vi "质控数据存储(子VI).vi"(4 "CODMn":refnum<vi>, 6 "总磷":refnum<vi>, 7 "CODCr":refnum<vi>, 10 "氨氮":refnum<vi>, 11 "总氮":refnum<vi>) -> ()   [LabVIEW 2016, in "质控单元.lvlib"]
uses:
  <vilib>/ptbypt/NI_PtbyPt.lvlib
panel:
  out "columns":string[](array[string])
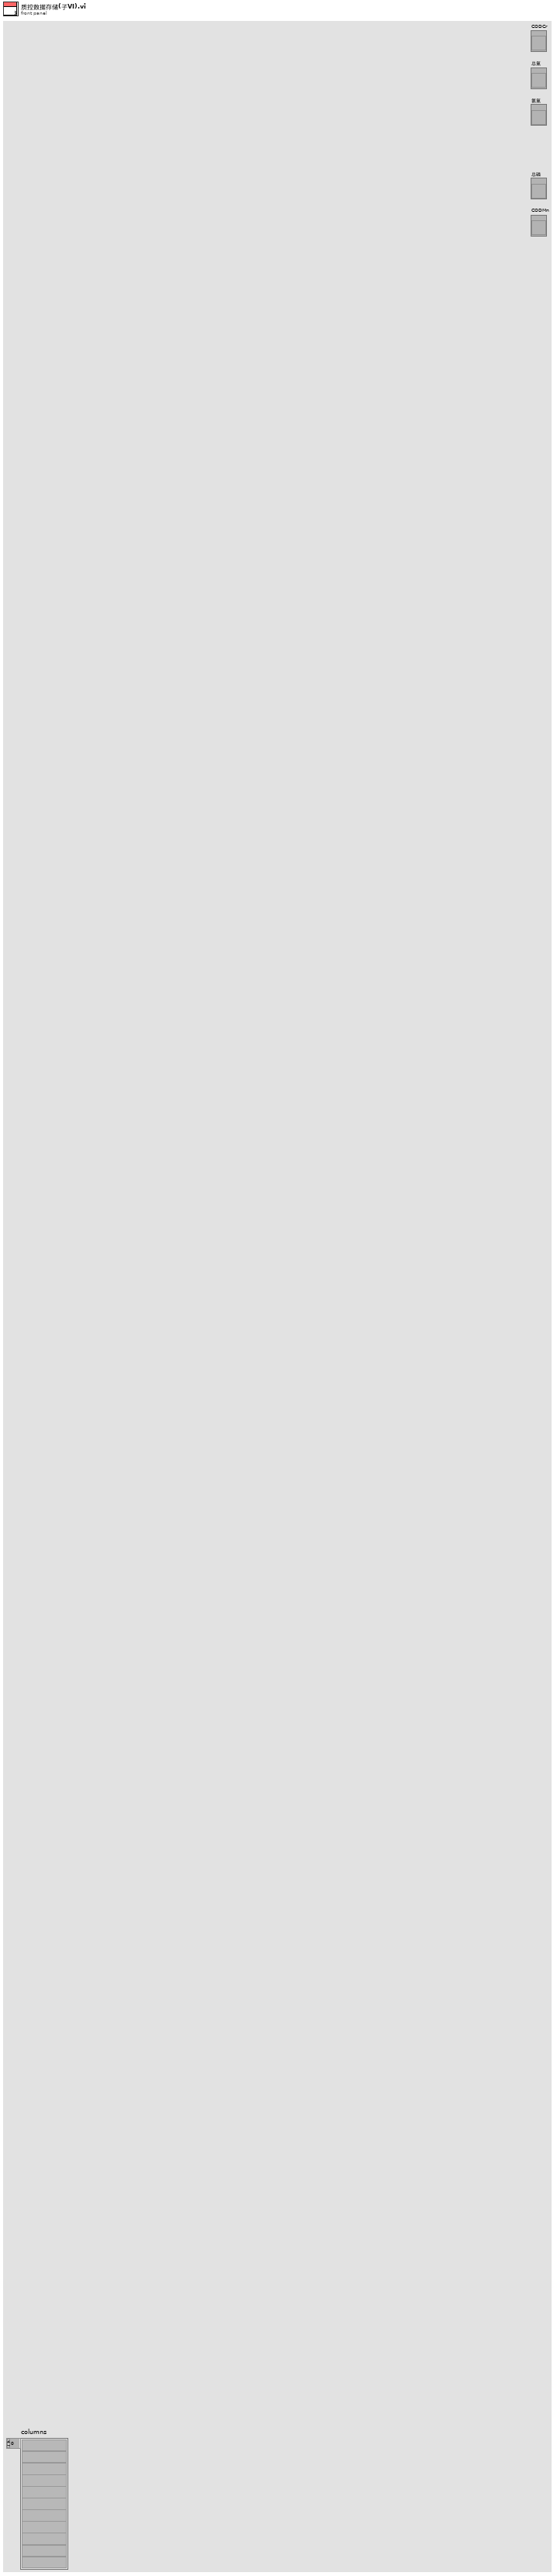
[diagram p1: front panel]
types:
  T1 = cluster{"时间":timestamp, "参数":string, "加标前水样测试时间":timestamp, "加标前水样浓度值（mg/L)":sgl, "加标后水样浓度值（mg/L)":sgl, "加标母液浓度值（mg/L)":sgl, "加标体积":dbl, "加标水杯定容体积":dbl, "加标回收率":dbl}
  T2 = cluster{"因子编码":u32, "单位":u16, "标样参考值":sgl, "水样数据时间":timestamp, "水样实测值":sgl, "水样数据标识":string, "标样数据时间":timestamp, "标样实测值":sgl, "标样数据标识":string, "空白数据时间":timestamp, "空白实测值":sgl, "空白数据标识":string, "零点核查数据时间":timestamp, "零点核查实测值":sgl, "零点核查数据标识":string, "跨度核查数据时间":timestamp, "跨度核查实测值":sgl, "跨度核查数据标识":string, "加标回收数据时间":timestamp, "加标回收实测值":sgl, "加标回收数据标识":string, "平行样数据时间":timestamp, "平行样实测值":sgl, "平行样数据标识":string}
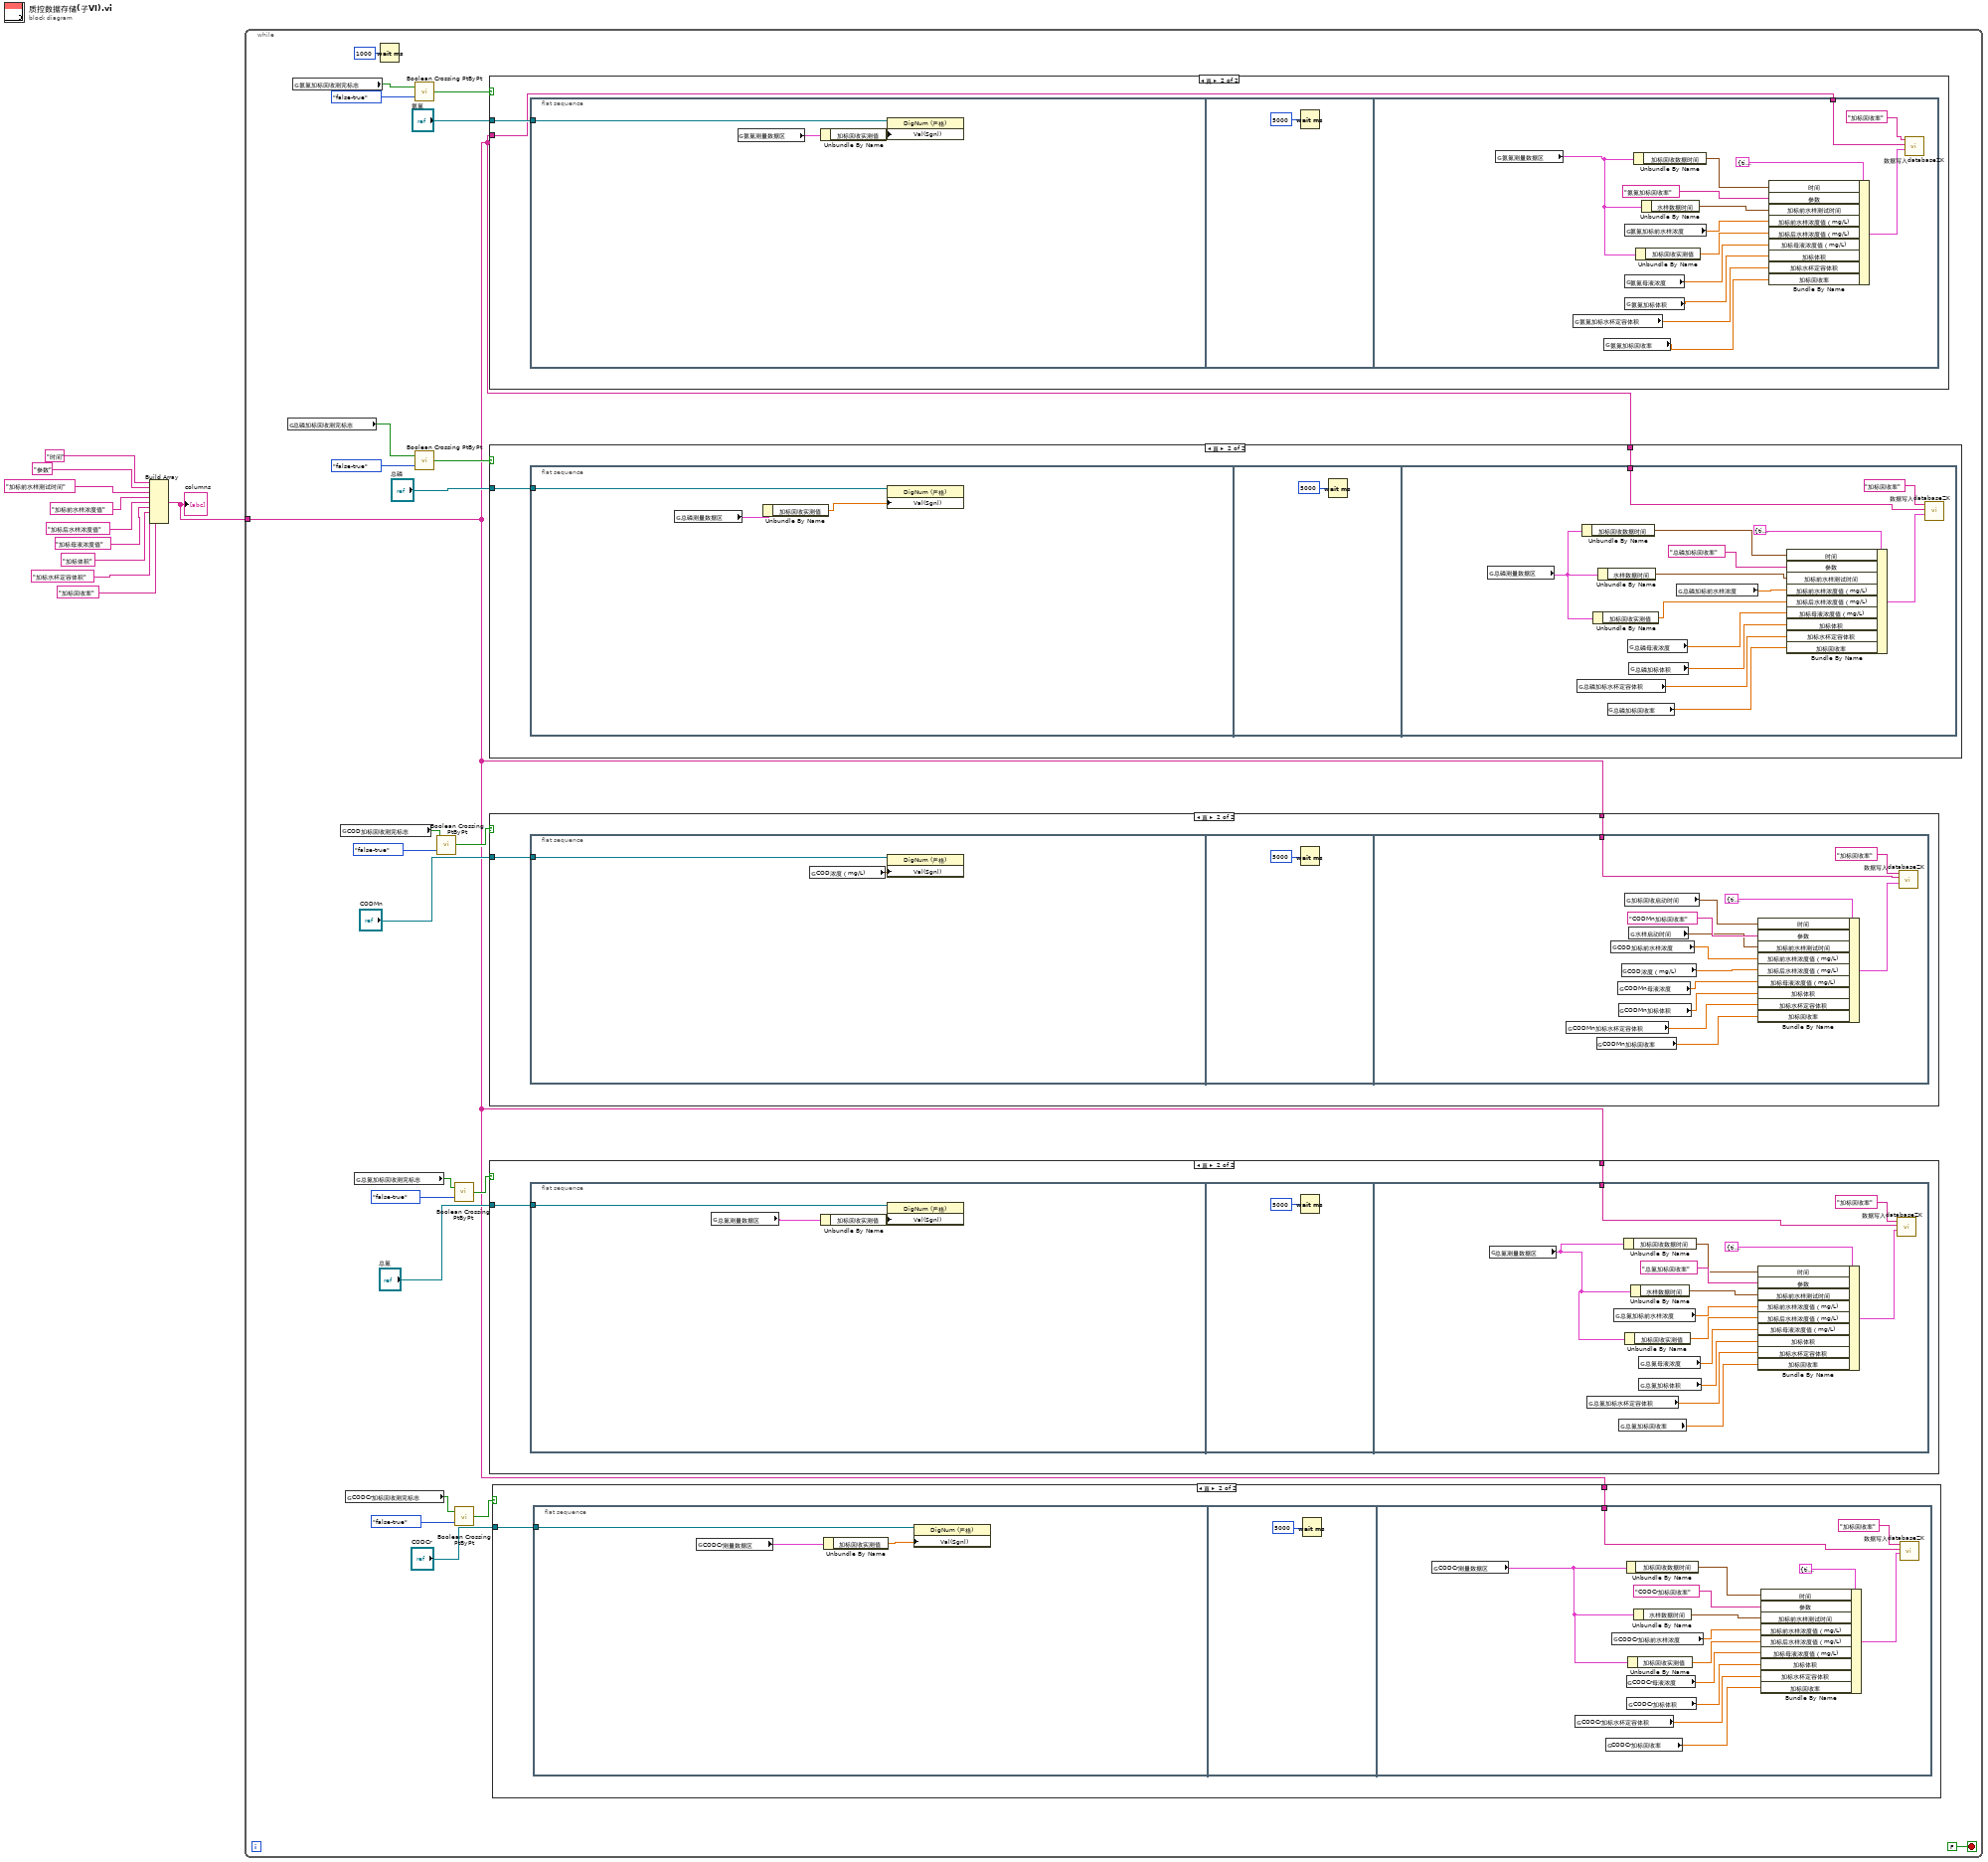
[diagram p0: block diagram]
diagram:
  n1 = Build Array("时间" ("table"), "参数" ("table"), "加标前水样测试时间" ("table"), "加标前水样浓度值" ("元素"), "加标后水样浓度值" ("元素"), "加标母液浓度值" ("元素"), "加标体积" ("元素"), "加标水杯定容体积" ("元素"), "加标回收率" ("元素")) -> (w1:string[])
  "columns" <- w1
  n2 = while {
    tunnel: w1 -> [w11]
    stop <- FALSE stop-if-true
    n3 = global read "质控测完标志全局 1.vi" "总磷加标回收测完标志"() -> (w24:bool)
    n4 = global read "质控测完标志全局 1.vi" "氨氮加标回收测完标志"() -> (w19:bool)
    n5 = global read "质控测完标志全局 1.vi" "COD加标回收测完标志"() -> (w26:bool)
    n6 = global read "质控测完标志全局 1.vi" "CODCr加标回收测完标志"() -> (w32:bool)
    n7 = global read "质控测完标志全局 1.vi" "总氮加标回收测完标志"() -> (w29:bool)
    n8 = Wait (ms)(milliseconds to wait=u32 1000 ("等待时间（毫秒）")) -> ()  [unwired: 1 out]
    n9 = call <vilib>:"Boolean Crossing PtByPt.vi"("direction"=enum16{"either", "false-true", "true-false"}."false-true", "input"=w19) -> ("crossing"=w20:bool)  [unwired: 1 in]
    n10 = call <vilib>:"Boolean Crossing PtByPt.vi"("direction"=enum16{"either", "false-true", "true-false"}."false-true", "input"=w24) -> ("crossing"=w23:bool)  [unwired: 1 in]
    n11 = call <vilib>:"Boolean Crossing PtByPt.vi"("direction"=enum16{"either", "false-true", "true-false"}."false-true", "input"=w26) -> ("crossing"=w27:bool)  [unwired: 1 in]
    n12 = call <vilib>:"Boolean Crossing PtByPt.vi"("direction"=enum16{"either", "false-true", "true-false"}."false-true", "input"=w29) -> ("crossing"=w30:bool)  [unwired: 1 in]
    n13 = call <vilib>:"Boolean Crossing PtByPt.vi"("direction"=enum16{"either", "false-true", "true-false"}."false-true", "input"=w32) -> ("crossing"=w33:bool)  [unwired: 1 in]
    n14 = case shown="真" w20 {
      tunnel: "氨氮" -> [_ w113]
      tunnel: w11 -> [_ w112]
      frame False {
      }
      frame True {
        n15 = flat-sequence {
          tunnel: w113 -> [w114]
          tunnel: w112 -> [w118]
          frame #0 {
            n16 = global read "与氨氮交互全局.vi" "氨氮测量数据区"() -> (w115:T2)
            n17 = Unbundle By Name(w115) -> ("加标回收实测值"=w116:sgl)
            n18 = property on="属性节点" class="DigNum (严格)"(reference=w114, "Val(Sgnl)"=w116) -> ()  [unwired: 1 in, 2 out]
          }
          frame #1 {
            n19 = Wait (ms)(milliseconds to wait=u32 5000 ("等待时间（毫秒）")) -> ()  [unwired: 1 out]
          }
          frame #2 {
            n20 = global read "与氨氮交互全局.vi" "氨氮测量数据区"() -> (w125:T2)
            n21 = global read "加标回收状态全局变量.vi" "氨氮加标水杯定容体积"() -> (w121:dbl)
            n22 = global read "加标回收状态全局变量.vi" "氨氮加标回收率"() -> (w122:dbl)
            n23 = global read "水样浓度全局.vi" "氨氮加标前水样浓度"() -> (w131:dbl)
            n24 = global read "加标回收状态全局变量.vi" "氨氮母液浓度"() -> (w119:dbl)
            n25 = global read "加标回收状态全局变量.vi" "氨氮加标体积"() -> (w120:dbl)
            n26 = Unbundle By Name(w125) -> ("加标回收数据时间"=w128:timestamp)
            n27 = Unbundle By Name(w125) -> ("加标回收实测值"=w130:sgl)
            n28 = Unbundle By Name(w125) -> ("水样数据时间"=w126:timestamp)
            n29 = Bundle By Name(cluster=T1 {"时间"=timestamp(0 s since 1904-01-01), "参数"="", "加标前水样测试时间"=timestamp(0 s since 1904-01-01), "加标前水样浓度值（mg/L)"=0.0, "加标后水样浓度值（mg/L)"=0.0, "加标母液浓度值（mg/L)"=0.0, "加标体积"=0.0, "加标水杯定容体积"=0.0, "加标回收率"=0.0} ("data"), "时间"=w128, "参数"="氨氮加标回收率" ("table"), "加标前水样测试时间"=w126, "加标前水样浓度值（mg/L)"=w131, "加标后水样浓度值（mg/L)"=w130, "加标母液浓度值（mg/L)"=w119, "加标体积"=w120, "加标水杯定容体积"=w121, "加标回收率"=w122) -> (w123:T1)
            n30 = call "数据写入databaseZK.vi"("data"=w123, "columns"=w118, "table"="加标回收率") -> ()  [unwired: 8 in, 1 out]
          }
        }
      }
    }
    n31 = case shown="真" w23 {
      tunnel: "总磷" -> [_ w93]
      tunnel: w11 -> [_ w92]
      frame False {
      }
      frame True {
        n32 = flat-sequence {
          tunnel: w93 -> [w94]
          tunnel: w92 -> [w98]
          frame #0 {
            n33 = global read "与总磷交互全局.vi" "总磷测量数据区"() -> (w95:T2)
            n34 = Unbundle By Name(w95) -> ("加标回收实测值"=w96:sgl)
            n35 = property on="属性节点" class="DigNum (严格)"(reference=w94, "Val(Sgnl)"=w96) -> ()  [unwired: 1 in, 2 out]
          }
          frame #1 {
            n36 = Wait (ms)(milliseconds to wait=u32 5000 ("等待时间（毫秒）")) -> ()  [unwired: 1 out]
          }
          frame #2 {
            n37 = global read "与总磷交互全局.vi" "总磷测量数据区"() -> (w105:T2)
            n38 = global read "加标回收状态全局变量.vi" "总磷加标水杯定容体积"() -> (w100:dbl)
            n39 = Unbundle By Name(w105) -> ("加标回收数据时间"=w108:timestamp)
            n40 = Unbundle By Name(w105) -> ("加标回收实测值"=w106:sgl)
            n41 = Unbundle By Name(w105) -> ("水样数据时间"=w107:timestamp)
            n42 = global read "加标回收状态全局变量.vi" "总磷加标回收率"() -> (w99:dbl)
            n43 = global read "加标回收状态全局变量.vi" "总磷母液浓度"() -> (w102:dbl)
            n44 = global read "加标回收状态全局变量.vi" "总磷加标体积"() -> (w101:dbl)
            n45 = global read "水样浓度全局.vi" "总磷加标前水样浓度"() -> (w111:dbl)
            n46 = Bundle By Name(cluster=T1 {"时间"=timestamp(0 s since 1904-01-01), "参数"="", "加标前水样测试时间"=timestamp(0 s since 1904-01-01), "加标前水样浓度值（mg/L)"=0.0, "加标后水样浓度值（mg/L)"=0.0, "加标母液浓度值（mg/L)"=0.0, "加标体积"=0.0, "加标水杯定容体积"=0.0, "加标回收率"=0.0} ("data"), "时间"=w108, "参数"="总磷加标回收率" ("table"), "加标前水样测试时间"=w107, "加标前水样浓度值（mg/L)"=w111, "加标后水样浓度值（mg/L)"=w106, "加标母液浓度值（mg/L)"=w102, "加标体积"=w101, "加标水杯定容体积"=w100, "加标回收率"=w99) -> (w103:T1)
            n47 = call "数据写入databaseZK.vi"("data"=w103, "columns"=w98, "table"="加标回收率") -> ()  [unwired: 8 in, 1 out]
          }
        }
      }
    }
    n48 = case shown="真" w27 {
      tunnel: "CODMn" -> [_ w75]
      tunnel: w11 -> [_ w74]
      frame False {
      }
      frame True {
        n49 = flat-sequence {
          tunnel: w75 -> [w76]
          tunnel: w74 -> [w79]
          frame #0 {
            n50 = global read "与CODMn交互全局.vi" "COD浓度（mg/L)"() -> (w77:dbl)
            n51 = property on="属性节点" class="DigNum (严格)"(reference=w76, "Val(Sgnl)"=w77) -> ()  [unwired: 1 in, 2 out]
          }
          frame #1 {
            n52 = Wait (ms)(milliseconds to wait=u32 5000 ("等待时间（毫秒）")) -> ()  [unwired: 1 out]
          }
          frame #2 {
            n53 = global read "加标回收状态全局变量.vi" "CODMn加标水杯定容体积"() -> (w81:dbl)
            n54 = global read "加标回收状态全局变量.vi" "CODMn加标回收率"() -> (w80:dbl)
            n55 = global read "水样浓度全局.vi" "COD加标前水样浓度"() -> (w91:dbl)
            n56 = global read "加标回收状态全局变量.vi" "CODMn母液浓度"() -> (w83:dbl)
            n57 = global read "加标回收状态全局变量.vi" "CODMn加标体积"() -> (w82:dbl)
            n58 = global read "与CODMn交互全局.vi" "COD浓度（mg/L)"() -> (w90:dbl)
            n59 = global read "与CODMn交互全局.vi" "加标回收启动时间"() -> (w87:timestamp)
            n60 = global read "与CODMn交互全局.vi" "水样启动时间"() -> (w86:timestamp)
            n61 = Bundle By Name(cluster=T1 {"时间"=timestamp(0 s since 1904-01-01), "参数"="", "加标前水样测试时间"=timestamp(0 s since 1904-01-01), "加标前水样浓度值（mg/L)"=0.0, "加标后水样浓度值（mg/L)"=0.0, "加标母液浓度值（mg/L)"=0.0, "加标体积"=0.0, "加标水杯定容体积"=0.0, "加标回收率"=0.0} ("data"), "时间"=w87, "参数"="CODMn加标回收率" ("table"), "加标前水样测试时间"=w86, "加标前水样浓度值（mg/L)"=w91, "加标后水样浓度值（mg/L)"=w90, "加标母液浓度值（mg/L)"=w83, "加标体积"=w82, "加标水杯定容体积"=w81, "加标回收率"=w80) -> (w84:T1)
            n62 = call "数据写入databaseZK.vi"("data"=w84, "columns"=w79, "table"="加标回收率") -> ()  [unwired: 8 in, 1 out]
          }
        }
      }
    }
    n63 = case shown="真" w30 {
      tunnel: "总氮" -> [_ w55]
      tunnel: w11 -> [_ w54]
      frame False {
      }
      frame True {
        n64 = flat-sequence {
          tunnel: w55 -> [w56]
          tunnel: w54 -> [w60]
          frame #0 {
            n65 = global read "与总氮交互全局.vi" "总氮测量数据区"() -> (w57:T2)
            n66 = Unbundle By Name(w57) -> ("加标回收实测值"=w58:sgl)
            n67 = property on="属性节点" class="DigNum (严格)"(reference=w56, "Val(Sgnl)"=w58) -> ()  [unwired: 1 in, 2 out]
          }
          frame #1 {
            n68 = Wait (ms)(milliseconds to wait=u32 5000 ("等待时间（毫秒）")) -> ()  [unwired: 1 out]
          }
          frame #2 {
            n69 = global read "与总氮交互全局.vi" "总氮测量数据区"() -> (w66:T2)
            n70 = global read "加标回收状态全局变量.vi" "总氮加标水杯定容体积"() -> (w62:dbl)
            n71 = global read "水样浓度全局.vi" "总氮加标前水样浓度"() -> (w73:dbl)
            n72 = global read "加标回收状态全局变量.vi" "总氮加标回收率"() -> (w61:dbl)
            n73 = Unbundle By Name(w66) -> ("加标回收数据时间"=w69:timestamp)
            n74 = Unbundle By Name(w66) -> ("加标回收实测值"=w72:sgl)
            n75 = Unbundle By Name(w66) -> ("水样数据时间"=w68:timestamp)
            n76 = global read "加标回收状态全局变量.vi" "总氮母液浓度"() -> (w64:dbl)
            n77 = global read "加标回收状态全局变量.vi" "总氮加标体积"() -> (w63:dbl)
            n78 = Bundle By Name(cluster=T1 {"时间"=timestamp(0 s since 1904-01-01), "参数"="", "加标前水样测试时间"=timestamp(0 s since 1904-01-01), "加标前水样浓度值（mg/L)"=0.0, "加标后水样浓度值（mg/L)"=0.0, "加标母液浓度值（mg/L)"=0.0, "加标体积"=0.0, "加标水杯定容体积"=0.0, "加标回收率"=0.0} ("data"), "时间"=w69, "参数"="总氮加标回收率" ("table"), "加标前水样测试时间"=w68, "加标前水样浓度值（mg/L)"=w73, "加标后水样浓度值（mg/L)"=w72, "加标母液浓度值（mg/L)"=w64, "加标体积"=w63, "加标水杯定容体积"=w62, "加标回收率"=w61) -> (w65:T1)
            n79 = call "数据写入databaseZK.vi"("data"=w65, "columns"=w60, "table"="加标回收率") -> ()  [unwired: 8 in, 1 out]
          }
        }
      }
    }
    n80 = case shown="真" w33 {
      tunnel: "CODCr" -> [_ w35]
      tunnel: w11 -> [_ w34]
      frame False {
      }
      frame True {
        n81 = flat-sequence {
          tunnel: w35 -> [w36]
          tunnel: w34 -> [w40]
          frame #0 {
            n82 = global read "与CODCr交互全局.vi" "CODCr测量数据区"() -> (w38:T2)
            n83 = Unbundle By Name(w38) -> ("加标回收实测值"=w37:sgl)
            n84 = property on="属性节点" class="DigNum (严格)"(reference=w36, "Val(Sgnl)"=w37) -> ()  [unwired: 1 in, 2 out]
          }
          frame #1 {
            n85 = Wait (ms)(milliseconds to wait=u32 5000 ("等待时间（毫秒）")) -> ()  [unwired: 1 out]
          }
          frame #2 {
            n86 = global read "与CODCr交互全局.vi" "CODCr测量数据区"() -> (w46:T2)
            n87 = global read "加标回收状态全局变量.vi" "CODCr加标水杯定容体积"() -> (w42:dbl)
            n88 = global read "加标回收状态全局变量.vi" "CODCr加标回收率"() -> (w41:dbl)
            n89 = global read "水样浓度全局.vi" "CODCr加标前水样浓度"() -> (w53:dbl)
            n90 = Unbundle By Name(w46) -> ("加标回收数据时间"=w49:timestamp)
            n91 = global read "加标回收状态全局变量.vi" "CODCr母液浓度"() -> (w44:dbl)
            n92 = global read "加标回收状态全局变量.vi" "CODCr加标体积"() -> (w43:dbl)
            n93 = Unbundle By Name(w46) -> ("加标回收实测值"=w52:sgl)
            n94 = Unbundle By Name(w46) -> ("水样数据时间"=w48:timestamp)
            n95 = Bundle By Name(cluster=T1 {"时间"=timestamp(0 s since 1904-01-01), "参数"="", "加标前水样测试时间"=timestamp(0 s since 1904-01-01), "加标前水样浓度值（mg/L)"=0.0, "加标后水样浓度值（mg/L)"=0.0, "加标母液浓度值（mg/L)"=0.0, "加标体积"=0.0, "加标水杯定容体积"=0.0, "加标回收率"=0.0} ("data"), "时间"=w49, "参数"="CODCr加标回收率" ("table"), "加标前水样测试时间"=w48, "加标前水样浓度值（mg/L)"=w53, "加标后水样浓度值（mg/L)"=w52, "加标母液浓度值（mg/L)"=w44, "加标体积"=w43, "加标水杯定容体积"=w42, "加标回收率"=w41) -> (w45:T1)
            n96 = call "数据写入databaseZK.vi"("data"=w45, "columns"=w40, "table"="加标回收率") -> ()  [unwired: 8 in, 1 out]
          }
        }
      }
    }
  }
